vi "ZNA_SettingMeas.vi"(4 "Mark_Freq(GHz)":dbl=39.0, 5 "Stop_Freq(GHz)":dbl=40.0, 6 "SweepPoints":i32=11, 7 "Start_Freq(GHz)":dbl=38.0, 8 "error in":errorcluster, 9 "sParameter":i32=21, 10 "Step_Freq(GHz)":dbl=0.5 format="%#_13g", 11 "VISA IN":refnum<visa-resource-name>="TCPIP0::192.168.100.12::inst0::INSTR") -> (0 "error out":errorcluster, 3 "Marker_array":dbl[](array[numeric]))   [LabVIEW 2023, in "R_S.lvlib"]
uses:
  R_S.lvlib
  CTL/RS_ZNA.ctl
panel:
  in  "Mark":i32=1
  in  "Meas":i32=1
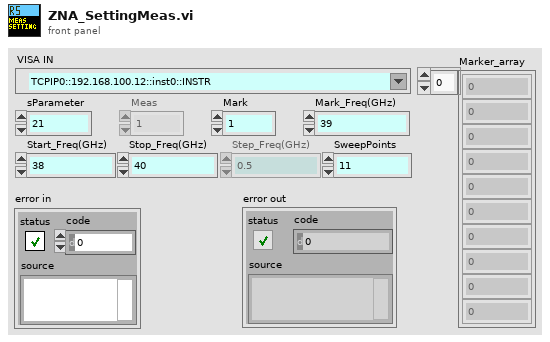
[diagram p1: front panel]
types:
  T1 = typedef "RS_ZNA.ctl" = enum16{"Init", "Close", "set_SweepPoint", "set_MeasFormat", "set_FreqStartStop", "set_MeasPAR_S", "set_MarkerON", "set_MarkerOFF", "set_MarkerFreq", "set_MarkerFormat", "set_TriggerSingle", "query_GainPhase"}
  T2 = cluster{"SweepPoints":i32, "StartFreq_GHz":dbl, "StopFreq_GHz":dbl, "S_Parameter":i32, "Marker_no.":i32, "Marker_Freq(GHz)":dbl}
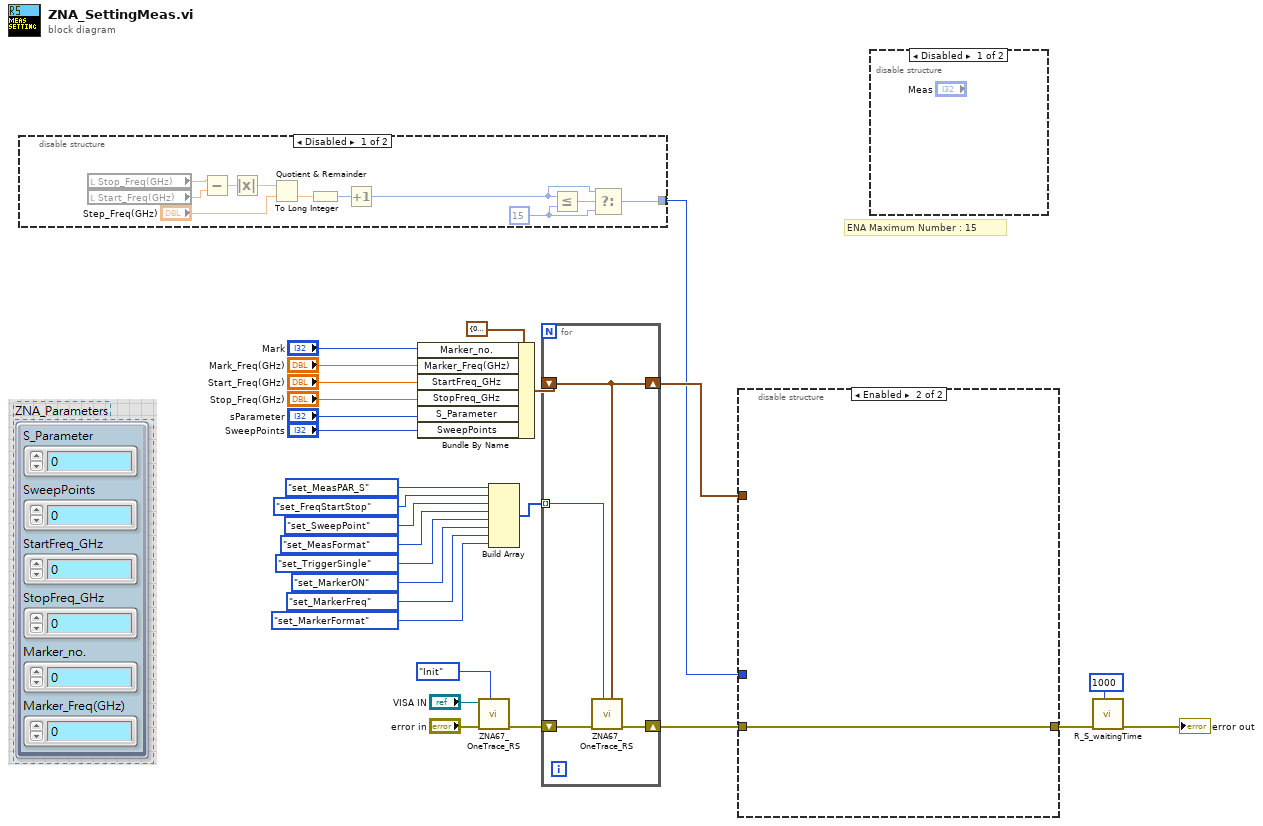
[diagram p0: block diagram]
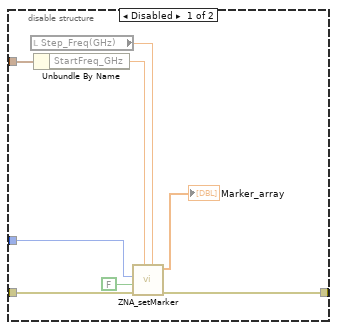
[diagram p3: hidden frame]
diagram:
  # "ENA Maximum Number : 15"
  n1 = disable-structure shown="Disabled" {
    disable-tunnel: [w28 _] -> w4
    frame Disabled {
      w30 = 15 ("y")
      n2 = local read "Stop_Freq(GHz)"() -> (w38:dbl)
      n3 = local read "Start_Freq(GHz)"() -> (w37:dbl)
      n4 = Subtract(x=w38, y=w37) -> (x-y=w36:dbl)
      n5 = Absolute Value(x=w36) -> (abs(x)=w34:dbl)
      n6 = Quotient & Remainder(x=w34, y="Step_Freq(GHz)") -> (floor(x/y)=w33:dbl)  [unwired: 1 out]
      n7 = To Long Integer(number=w33) -> (32bit integer=w32:i32)
      n8 = Increment(x=w32) -> (x+1=w29:i32)
      n9 = Less Or Equal?(x=w29, y=w30) -> (x <= y?=w31:bool)
      n10 = Select(t=w29, s=w31, f=w30) -> (s? t:f=w28:i32)
    }
    frame Enabled {
    }
  }
  n11 = Bundle By Name(cluster=T2 {"SweepPoints"=0, "StartFreq_GHz"=0.0, "StopFreq_GHz"=0.0, "S_Parameter"=0, "Marker_no."=0, "Marker_Freq(GHz)"=0.0} ("ZNA_Parameters 2"), "Marker_no."="Mark", "Marker_Freq(GHz)"="Mark_Freq(GHz)", "StartFreq_GHz"="Start_Freq(GHz)", "StopFreq_GHz"="Stop_Freq(GHz)", "S_Parameter"="sParameter", "SweepPoints"="SweepPoints") -> (w7:T2)
  n12 = call "ZNA67_OneTrace_RS.vi"("ZNA_Func."=RS_ZNA."Init", "error in"="error in", "VISA IN"="VISA IN") -> ("error out"=w24:errorcluster)  [unwired: 5 in, 3 out]
  n13 = Build Array(RS_ZNA."set_MeasPAR_S" ("ZNA_Func."), RS_ZNA."set_FreqStartStop" ("ZNA_Func."), RS_ZNA."set_SweepPoint" ("ZNA_Func."), RS_ZNA."set_MeasFormat" ("ZNA_Func."), RS_ZNA."set_TriggerSingle" ("ZNA_Func."), RS_ZNA."set_MarkerON" ("ZNA_Func."), RS_ZNA."set_MarkerFreq" ("ZNA_Func."), RS_ZNA."set_MarkerFormat" ("ZNA_Func.")) -> (w16:T1[])
  n14 = for {
    shift-right: [w39] -> w6
    shift-left: w7 -> [w39]
    shift-right: [w41] -> w14
    shift-left: w24 -> [w42]
    tunnel: w16 -> [w40] mode=indexing
    n15 = call "ZNA67_OneTrace_RS.vi"("ZNA_Parameters"=w39, "ZNA_Func."=w40, "error in"=w42) -> ("error out"=w41:errorcluster)  [unwired: 5 in, 3 out]
  }
  n16 = disable-structure shown="Enabled" {
    disable-tunnel: w14 -> [w50 w51]
    disable-tunnel: [w49 w51] -> w13
    disable-tunnel: w6 -> [w44 _]
    disable-tunnel: w4 -> [w43 _]
    frame Disabled {
      n17 = local read "Step_Freq(GHz)"() -> (w47:dbl)
      n18 = Unbundle By Name(w44) -> ("StartFreq_GHz"=w48:dbl)
      n19 = call "ZNA_setMarker.vi"("Step_Freq(GHz)"=w47, "Start_Freq(GHz)"=w48, "error in"=w50, "Simulation"=FALSE, "Markers_num"=w43) -> ("error out"=w49:errorcluster, "Marker_array"=→"Marker_array":dbl[])  [unwired: 5 in]
    }
    frame Enabled {
    }
  }
  n20 = disable-structure shown="Disabled" {
    frame Disabled {
    }
    frame Enabled {
    }
  }
  n21 = call "R_S_waitingTime.vi"("Waiting Time(ms)"=u32 1000, "error in"=w13) -> ("error out"=→"error out":errorcluster)  [unwired: 9 in]
